vi "DefaultFromIni.vi"(8 "error in (no error)":errorcluster, 11 "NiPxi6123 in":refnum<class "NiPxi6123.lvclass">) -> (0 "error out":errorcluster, 3 "NiPxi6123 out":refnum<class "NiPxi6123.lvclass">)   [LabVIEW 2014, in "SamplerPlugins.lvlib" / "NiPxi6123.lvclass"]
uses:
  NiPxi6123.lvclass
  NiBaseClass/NiBase.lvclass
  <vilib>/Utility/config.llb/NI_LVConfig.lvlib
  TypeDefs/eSampleMode.ctl
  <vilib>/Utility/error.llb/Error Cluster From Error Code.vi
  <vilib>/ErrorRing/Error Ring.xnode
  TypeDefs/sPhysicalChannels.ctl
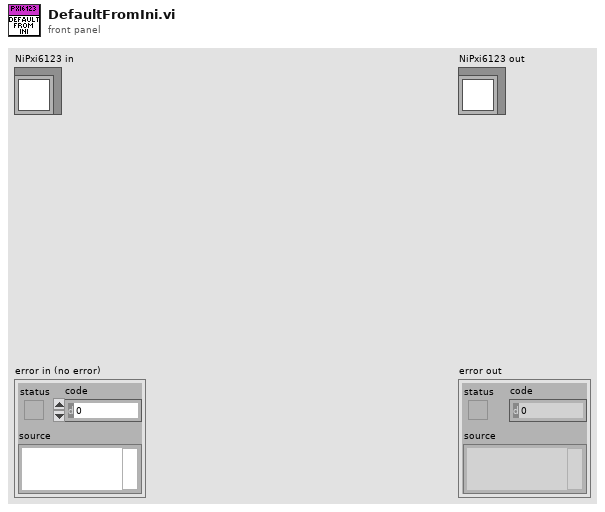
[diagram p1: front panel]
types:
  T1 = typedef "SamplerPlugins.lvlib/NiPxi6123.lvclass/eSampleMode.ctl" = i32
  T2 = typedef "SamplerPlugins.lvlib/NiPxi6123.lvclass/sPhysicalChannels.ctl" = string[]
  T3 = typedef "NI_LVConfig.lvlib/Config Data RefNum.ctl" = refnum<k1>
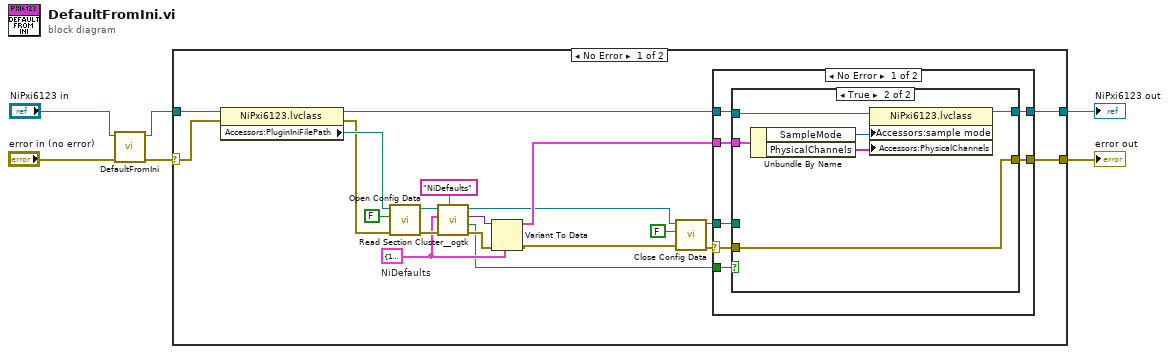
[diagram p0: block diagram]
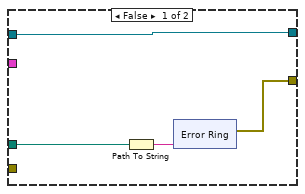
[diagram p2: hidden frame]
diagram:
  n1 = call-parent "DefaultFromIni.vi"("error in (no error)"="error in (no error)", "SamplerPluginsBase in"="NiPxi6123 in") -> ("error out"=w2:errorcluster, "SamplerPluginsBase out"=w6:refnum<class "NiPxi6123.lvclass">)  [unwired: 8 in]
  n2 = case shown="No Error" w2 {
    selector: w2 -> [w25 w55]
    tunnel: w6 -> [w27 w54]
    tunnel: [w20 w54] -> w3
    tunnel: [w18 w55] -> w1
    frame No Error {
      w10 = cluster{"SampleMode":T1, "PhysicalChannels":T2} {"SampleMode"=10123, "PhysicalChannels"=["", "", "", "", "", "", "", "", ""]}  # NiDefaults
      n3 = property class="NiPxi6123.lvclass"(reference=w27, error in=w25) -> (reference out=w26:refnum<class "NiPxi6123.lvclass">, error out=w22:errorcluster, "Accessors:PluginIniFilePath"=w24:path)
      n4 = call <vilib>:"Open Config Data.vi"("error in (no error)"=w22, "create file if necessary (T)"=FALSE, "configuration file path"=w24) -> ("error out"=w11:errorcluster, "refnum"=w12:T3)  [unwired: 6 in, 1 out]
      n5 = call <userlib>:"Read Section Cluster__ogtk.vi"("section (optional)"="NiDefaults" ("section"), "error in (no error)"=w11, "Section Formatted Cluster Type"=w10, "refnum"=w12) -> ("error out"=w21:errorcluster, "all found?"=w9:bool, "Section Formatted Cluster"=w14:variant, "dup refnum"=w8:T3)  [unwired: 3 in, 1 out]
      n6 = Variant To Data(error in=w21, type=w10, Variant=w14) -> (data=w19:cluster{"SampleMode":T1, "PhysicalChannels":T2}, error out=w7:errorcluster)
      n7 = call <vilib>:"Close Config Data.vi"("error in (no error)"=w7, "write file if changed (T)"=FALSE, "refnum"=w8) -> ("error out"=w17:errorcluster, "file path"=w16:path)  [unwired: 7 in]
      n8 = case shown="No Error" w17 {
        selector: w17 -> [w29 w53]
        tunnel: w26 -> [w34 w52]
        tunnel: [w33 w52] -> w20
        tunnel: w19 -> [w32 _]
        tunnel: [w31 w53] -> w18
        tunnel: w9 -> [w30 _]
        tunnel: w16 -> [w28 _]
        frame No Error {
          n9 = case shown="True" w30 {
            tunnel: w34 -> [w35 w51]
            tunnel: [w35 w50] -> w33
            tunnel: w32 -> [_ w47]
            tunnel: [w36 w46] -> w31
            tunnel: w29 -> [_ w46]
            tunnel: w28 -> [w38 _]
            frame False {
              n10 = Path To String(path=w38) -> (string=w37:string)
              n11 = xnode "Error Ring"("parameter 0"=w37) -> ("error out"=w36:errorcluster)
            }
            frame True {
              n12 = Unbundle By Name(w47) -> ("SampleMode"=w48:T1, "PhysicalChannels"=w49:T2)
              n13 = property class="NiPxi6123.lvclass"(reference=w51, "Accessors:sample mode"=w48, "Accessors:PhysicalChannels"=w49) -> (reference out=w50:refnum<class "NiPxi6123.lvclass">)  [unwired: 1 in, 1 out]
            }
          }
        }
        frame Error {
        }
      }
    }
    frame Error {
    }
  }
  "error out" <- w1
  "NiPxi6123 out" <- w3
